vi "Action.vi"(8 "error in (no error)":errorcluster, 11 "GPackCLI in":refnum<class "GPackCLI.lvclass">) -> (0 "error out":errorcluster, 3 "GPackCLI out":refnum<class "GPackCLI.lvclass">)   [LabVIEW 2020, in "GPackTools.lvlib" / "GPackCLI.lvclass"]
uses:
  GPackCLI.lvclass
  GPackCLI.lvclass/GPackCLI.ctl
  GPack/Package/Package.lvclass
  GPack/PackageAbstract/PackageAbstract.lvclass
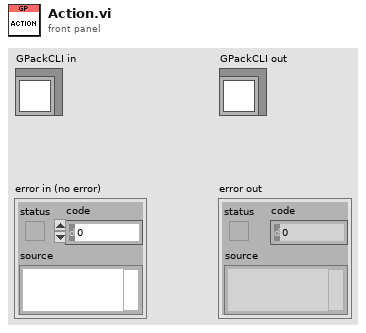
[diagram p1: front panel]
types:
  T1 = typedef "GPackTools.lvlib/GPackCLI.lvclass/Action.ctl" = enum16{"init", "install", "update", "addproj"}
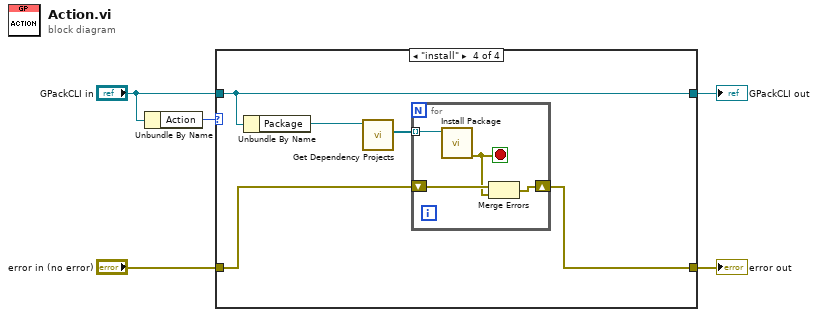
[diagram p0: block diagram]
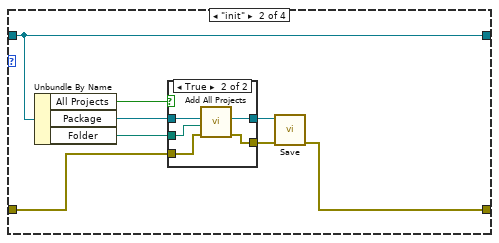
[diagram p3: hidden frame]
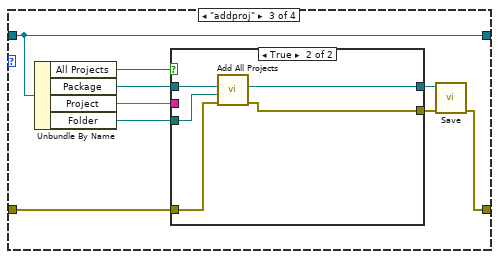
[diagram p5: hidden frame]
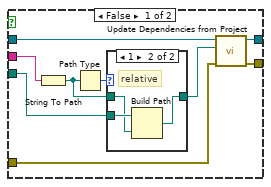
[diagram p6: hidden frame]
diagram:
  n1 = Unbundle By Name("GPackCLI in") -> ("Action"=w5:T1)
  n2 = case shown="\"install\"" w5 {
    tunnel: "GPackCLI in" -> [w7 w15 w31 w54]
    tunnel: "error in (no error)" -> [w6 w12 w26 w51]
    tunnel: [w6 w8 w30 w50] -> w2
    tunnel: [w7 w15 w31 w54] -> w1
    frame Default {
    }
    frame "init" {
      n3 = Unbundle By Name(w15) -> ("All Projects"=w14:bool, "Package"=w13:refnum<class "PackageAbstract.lvclass">, "Folder"=w11:path)
      n4 = case shown="True" w14 {
        tunnel: w13 -> [w16 w22]
        tunnel: w12 -> [w17 w20]
        tunnel: w11 -> [_ w21]
        tunnel: [w17 w19] -> w9
        tunnel: [w16 w18] -> w10
        frame False {
        }
        frame True {
          n5 = call "Add All Projects.vi"("error in (no error)"=w20, "Folder"=w21, "GPack.lvlib:PackageAbstract.lvclass in"=w22) -> ("error out"=w19:errorcluster, "GPack.lvlib:PackageAbstract.lvclass out"=w18:refnum<class "PackageAbstract.lvclass">)  [unwired: 7 in]
        }
      }
      n6 = call "Save.vi"("error in (no error)"=w9, "PackageAbstract in"=w10) -> ("error out"=w8:errorcluster)  [unwired: 8 in, 1 out]
    }
    frame "addproj" {
      n7 = Unbundle By Name(w31) -> ("All Projects"=w23:bool, "Package"=w27:refnum<class "PackageAbstract.lvclass">, "Project"=w29:string, "Folder"=w28:path)
      n8 = case shown="True" w23 {
        tunnel: w29 -> [w40 _]
        tunnel: w28 -> [w37 w48]
        tunnel: w27 -> [w36 w49]
        tunnel: w26 -> [w34 w47]
        tunnel: [w33 w45] -> w25
        tunnel: [w32 w46] -> w24
        frame False {
          n9 = String To Path(string=w40) -> (path=w38:path)
          n10 = Path Type(1:w38) -> (0:w39:i16)
          n11 = case shown="1" w39 {
            tunnel: w38 -> [w41 w43]
            tunnel: [w41 w42] -> w35
            tunnel: w37 -> [_ w44]
            frame 0, Default {
              # "Absolute"
            }
            frame 1 {
              # "relative"
              n12 = Build Path(base path=w44, name or relative path=w43) -> (appended path=w42:path)
            }
          }
          n13 = call "Update Dependencies from Project.vi"("error in (no error)"=w34, "lvproj Path"=w35, "PackageAbstract in"=w36) -> ("error out"=w33:errorcluster, "PackageAbstract out"=w32:refnum<class "PackageAbstract.lvclass">)  [unwired: 7 in]
        }
        frame True {
          n14 = call "Add All Projects.vi"("error in (no error)"=w47, "Folder"=w48, "GPack.lvlib:PackageAbstract.lvclass in"=w49) -> ("error out"=w45:errorcluster, "GPack.lvlib:PackageAbstract.lvclass out"=w46:refnum<class "PackageAbstract.lvclass">)  [unwired: 7 in]
        }
      }
      n15 = call "Save.vi"("error in (no error)"=w25, "PackageAbstract in"=w24) -> ("error out"=w30:errorcluster)  [unwired: 8 in, 1 out]
    }
    frame "install" {
      n16 = Unbundle By Name(w54) -> ("Package"=w53:refnum<class "PackageAbstract.lvclass">)
      n17 = call "Get Dependency Projects.vi"("PackageAbstract in"=w53) -> ("Dependencies"=w52:refnum<class "Package.lvclass">[])  [unwired: 8 in, 2 out]
      n18 = for {
        tunnel: w52 -> [w58] mode=indexing
        shift-right: [w56] -> w50
        shift-left: w51 -> [w57]
        stop <- w55 stop-if-true
        n19 = call-dynamic "Install Package.vi"("Package in"=w58) -> ("error out"=w55:errorcluster)  [unwired: 9 in, 1 out]
        n20 = Merge Errors(w57, w55) -> (w56:errorcluster)
      }
    }
  }
  "error out" <- w2
  "GPackCLI out" <- w1
